vi "padstringzero.vi"(1 "Length":i32, 2 "str":string="0") -> (0 "res":string="0")   [LabVIEW 2013]
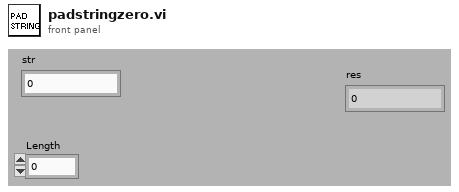
[diagram p1: front panel]
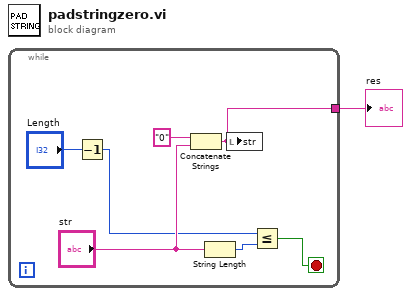
[diagram p0: block diagram]
diagram:
  n1 = while {
    tunnel: [w7] -> w1
    stop <- w2 stop-if-true
    n2 = Decrement(x="Length") -> (x-1=w4:i32)
    n3 = Concatenate Strings("0", "str") -> (w7:string)
    n4 = String Length(string="str") -> (length=w3:i32)
    n5 = local write "str"(w7) -> ()
    n6 = Less Or Equal?(x=w4, y=w3) -> (x <= y?=w2:bool)
  }
  "res" <- w1
